vi "Full Force Test.vi"(8 "error in (no error)":errorcluster, 10 "Model in":refnum<class "Model.lvclass">, 11 "Test Actuator State in":refnum<class "Test Actuator State.lvclass">) -> (0 "error out":errorcluster, 2 "Model out":refnum<class "Model.lvclass">, 3 "Test Actuator State out":refnum<class "Test Actuator State.lvclass">)   [LabVIEW 2015, in "Test Actuator State.lvclass"]
uses:
  Test Actuator State.lvclass
  Model/Model/Model.lvclass
  Model/Model/Model.lvclass/Model.ctl
  Typedefs/ActuatorSetPoints.ctl
  Typedefs/FAMT Typedefs.lvlib
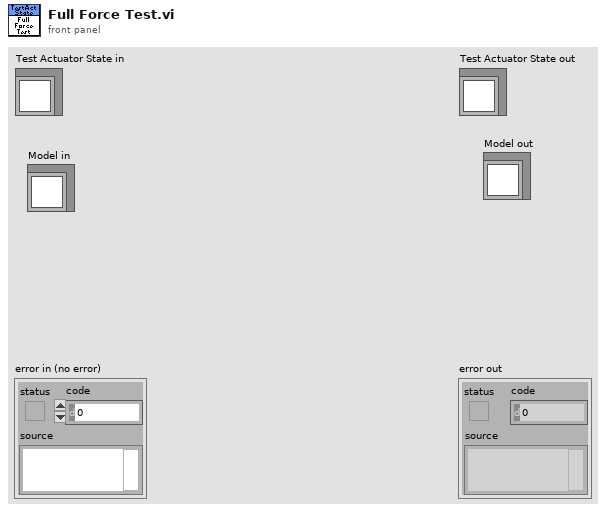
[diagram p1: front panel]
types:
  T1 = typedef "FAMT Typedefs.lvlib/FullForceScanSettings.ctl" = cluster{"Axial Force 1":dbl, "Lateral Force 1":dbl, "Axial Force 2":dbl, "Lateral Force 2":dbl, "Axial Force 3":dbl, "Lateral Force 3":dbl, "Axial Force 4":dbl, "Lateral Force 4":dbl, "Sample Time":dbl, "Process Time":dbl, "Tolerance %":dbl}
  T2 = cluster{"Axial Force 1":dbl, "Lateral Force 1":dbl}
  T3 = cluster{"Axial Force 2":dbl, "Lateral Force 2":dbl}
  T4 = cluster{"Axial Force 3":dbl, "Lateral Force 3":dbl}
  T5 = cluster{"Axial Force 4":dbl, "Lateral Force 4":dbl}
  T6 = cluster{"Axial Force 4":dbl, "Lateral Force 4":dbl}[]
  T7 = typedef "FAMT Typedefs.lvlib/ActuatorSetPoints.ctl" = cluster{"Axial Force":dbl, "Lateral Force":dbl, "FC1 Force":dbl, "FC2 Force":dbl}
  T8 = typedef "FAMT Typedefs.lvlib/ActuatorData.ctl" = cluster{"Timestamp":dbl, "Axial Force":dbl, "Lateral Force":dbl, "FC1 Force":dbl, "FC2 Force":dbl, "Lateral Push Pressure":dbl, "Lateral Pull Pressure":dbl, "Axial Push Pressure":dbl, "Axial Pull Pressure":dbl}
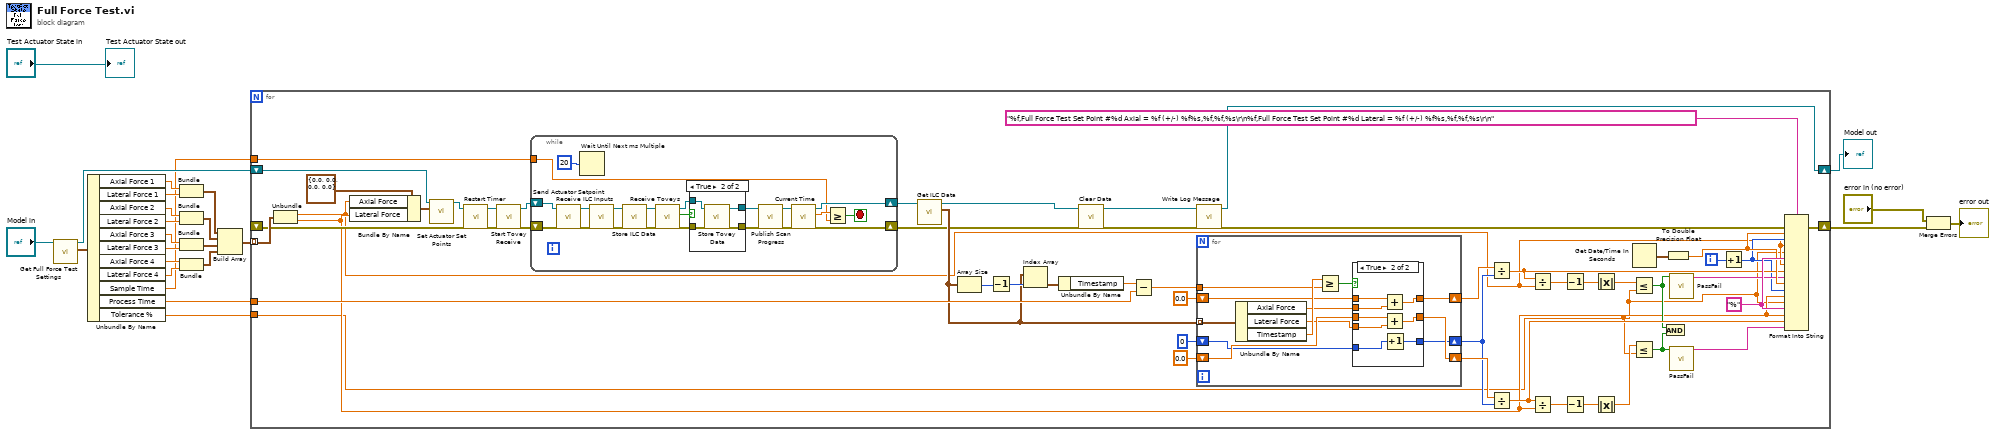
[diagram p0: block diagram]
diagram:
  n1 = call "Get Full Force Test Settings.vi"("Model in"="Model in") -> ("Full Force Test Settings"=w22:T1, "Model out"=w8:refnum<class "Model.lvclass">)  [unwired: 9 in]
  n2 = Unbundle By Name(w22) -> ("Axial Force 1"=w21:dbl, "Lateral Force 1"=w20:dbl, "Axial Force 2"=w18:dbl, "Lateral Force 2"=w17:dbl, "Axial Force 3"=w15:dbl, "Lateral Force 3"=w14:dbl, "Axial Force 4"=w12:dbl, "Lateral Force 4"=w11:dbl, "Sample Time"=w7:dbl, "Process Time"=w6:dbl, "Tolerance %"=w5:dbl)
  n3 = Bundle("Axial Force 1"=w21, "Lateral Force 1"=w20) -> (w19:T2)  [unwired: 1 in]
  n4 = Bundle("Axial Force 2"=w18, "Lateral Force 2"=w17) -> (w16:T3)  [unwired: 1 in]
  n5 = Bundle("Axial Force 3"=w15, "Lateral Force 3"=w14) -> (w13:T4)  [unwired: 1 in]
  n6 = Bundle("Axial Force 4"=w12, "Lateral Force 4"=w11) -> (w10:T5)  [unwired: 1 in]
  n7 = Build Array(w19, w16, w13, w10) -> (w9:T6)
  n8 = for {
    tunnel: w9 -> [w76] mode=indexing
    shift-right: [w49] -> w2
    shift-left: w8 -> [w75]
    tunnel: w7 -> [w74]
    tunnel: w6 -> [w68]
    tunnel: w5 -> [w31]
    shift-right: [w36] -> w1
    shift-left: _ -> [w51]
    i -> [w35]
    w45 = "%"
    n9 = Unbundle(w76) -> ("Axial Force 4"=w32:dbl, "Lateral Force 4"=w33:dbl)
    n10 = Bundle By Name(cluster=T7 {"Axial Force"=0.0, "Lateral Force"=0.0, "FC1 Force"=0.0, "FC2 Force"=0.0} ("Actuator Set Points"), "Axial Force"=w32, "Lateral Force"=w33) -> (w25:T7)
    n11 = call "Set Actuator Set Points.vi"("Actuator Set Points"=w25, "Model in"=w75) -> ("Model out"=w26:refnum<class "Model.lvclass">)  [unwired: 9 in]
    n12 = call "Restart Timer.vi"("error in (no error)"=w51, "Model in"=w26) -> ("error out"=w29:errorcluster, "Model out"=w30:refnum<class "Model.lvclass">)  [unwired: 8 in]
    n13 = call "Start Tovey Receive.vi"("error in (no error)"=w29, "Model in"=w30) -> ("error out"=w27:errorcluster, "Model out"=w28:refnum<class "Model.lvclass">)  [unwired: 8 in]
    n14 = while {
      shift-right: [w114] -> w73
      shift-left: w28 -> [w120]
      shift-right: [w113] -> w52
      shift-left: w27 -> [w117]
      tunnel: w74 -> [w111]
      stop <- w110 stop-if-true
      n15 = call "Send Actuator Setpoint.vi"("error in (no error)"=w117, "Model in"=w120) -> ("error out"=w116:errorcluster, "Model out"=w119:refnum<class "Model.lvclass">)  [unwired: 8 in]
      n16 = Wait Until Next ms Multiple(millisecond multiple=u32 20) -> ()  [unwired: 1 out]
      n17 = call "Receive ILC Inputs.vi"("error in (no error)"=w116, "Model in"=w119) -> ("error out"=w115:errorcluster, "Model out"=w118:refnum<class "Model.lvclass">)  [unwired: 8 in]
      n18 = call "Store ILC Data.vi"("error in (no error)"=w115, "Model in"=w118) -> ("error out"=w108:errorcluster, "Model out"=w109:refnum<class "Model.lvclass">)  [unwired: 8 in]
      n19 = call "Receive Toveys.vi"("error in (no error)"=w108, "Model in"=w109) -> ("error out"=w106:errorcluster, "Data Received"=w105:bool, "Model out"=w107:refnum<class "Model.lvclass">)  [unwired: 7 in]
      n20 = case shown="True" w105 {
        tunnel: w107 -> [w123 w127]
        tunnel: w106 -> [w122 w126]
        tunnel: [w122 w125] -> w101
        tunnel: [w123 w124] -> w104
        frame False {
        }
        frame True {
          n21 = call "Store Tovey Data.vi"("error in (no error)"=w126, "Model in"=w127) -> ("error out"=w125:errorcluster, "Model out"=w124:refnum<class "Model.lvclass">)  [unwired: 8 in]
        }
      }
      n22 = call "Publish Scan Progress.vi"("error in (no error)"=w101, "Model in"=w104) -> ("error out"=w102:errorcluster, "Model out"=w103:refnum<class "Model.lvclass">)  [unwired: 8 in]
      n23 = call "Current Time.vi"("error in (no error)"=w102, "Model in"=w103) -> ("error out"=w113:errorcluster, "Time"=w112:dbl, "Model out"=w114:refnum<class "Model.lvclass">)  [unwired: 7 in]
      n24 = Greater Or Equal?(x=w112, y=w111) -> (x >= y?=w110:bool)
    }
    n25 = call "Get ILC Data.vi"("Model in"=w73) -> ("ILCData"=w67:T8[], "Model out"=w53:refnum<class "Model.lvclass">)  [unwired: 9 in]
    n26 = Array Size(array=w67) -> (size(s)=w72:i32)
    n27 = Decrement(x=w72) -> (x-1=w71:i32)
    n28 = Index Array(array=w67, index=w71) -> (element=w70:T8)
    n29 = Unbundle By Name(w70) -> ("Timestamp"=w69:dbl)
    n30 = call "Clear Data.vi"("error in (no error)"=w52, "Model in"=w53) -> ("error out"=w48:errorcluster, "Model out"=w50:refnum<class "Model.lvclass">)  [unwired: 8 in]
    n31 = Subtract(x=w69, y=w68) -> (x-y=w66:dbl)
    n32 = call "Write Log Message.vi"("error in (no error)"=w48, "Model in"=w50) -> ("error out"=w37:errorcluster, "Model out"=w49:refnum<class "Model.lvclass">)  [unwired: 8 in]
    n33 = for {
      tunnel: w67 -> [w89] mode=indexing
      tunnel: w66 -> [w87]
      shift-right: [w84] -> w62
      shift-left: 0.0 -> [w86]
      shift-right: [w81] -> w61
      shift-left: 0.0 -> [w83]
      shift-right: [w78] -> w60
      shift-left: 0 -> [w79]
      n34 = Unbundle By Name(w89) -> ("Axial Force"=w85:dbl, "Lateral Force"=w82:dbl, "Timestamp"=w88:dbl)
      n35 = Greater Or Equal?(x=w88, y=w87) -> (x >= y?=w80:bool)
      n36 = case shown="True" w80 {
        tunnel: w86 -> [w91 w100]
        tunnel: w85 -> [_ w99]
        tunnel: [w91 w98] -> w84
        tunnel: w83 -> [w92 w97]
        tunnel: w82 -> [_ w96]
        tunnel: [w92 w95] -> w81
        tunnel: w79 -> [w90 w94]
        tunnel: [w90 w93] -> w78
        frame False {
        }
        frame True {
          n37 = Add(x=w100, y=w99) -> (x+y=w98:dbl)
          n38 = Add(x=w97, y=w96) -> (x+y=w95:dbl)
          n39 = Increment(x=w94) -> (x+1=w93:i32)
        }
      }
    }
    n40 = Divide(x=w62, y=w60) -> (x/y=w43:dbl)
    n41 = Divide(x=w61, y=w60) -> (x/y=w42:dbl)
    n42 = Divide(x=w43, y=w32) -> (x/y=w59:dbl)
    n43 = Divide(x=w42, y=w33) -> (x/y=w58:dbl)
    n44 = Decrement(x=w59) -> (x-1=w57:dbl)
    n45 = Decrement(x=w58) -> (x-1=w56:dbl)
    n46 = Absolute Value(x=w57) -> (abs(x)=w55:dbl)
    n47 = Absolute Value(x=w56) -> (abs(x)=w54:dbl)
    n48 = Less Or Equal?(x=w55, y=w31) -> (x <= y?=w41:bool)
    n49 = Less Or Equal?(x=w54, y=w31) -> (x <= y?=w39:bool)
    n50 = Get Date/Time In Seconds() -> (seconds since 1Jan1904=w46:timestamp)
    n51 = And(x=w41, y=w39) -> ()  [unwired: 1 out]
    n52 = To Double Precision Float(number=w46) -> (double precision float=w44:dbl)
    n53 = call "PassFail.vi"("Pass?"=w41) -> ("Result"=w40:string)  [unwired: 10 in]
    n54 = call "PassFail.vi"("Pass?"=w39) -> ("Result"=w38:string)  [unwired: 10 in]
    n55 = Increment(x=w35) -> (x+1=w34:i32)
    n56 = Format Into String(format string="%f,Full Force Test Set Point #%d Axial = %f (+/-) %f%s,%f,%f,%s\r\n%f,Full Force Test Set Point #%d Lateral = %f (+/-) %f%s,%f,%f,%s\r\n", error in=w37, w44, w34, w32, w31, w45, w32, w43, w40, w44, w34, w33, w31, w45, w33, w42, w38) -> (error out=w36:errorcluster)  [unwired: 1 in, 1 out]
  }
  "Model out" <- w2
  n57 = Merge Errors("error in (no error)", w1) -> (→"error out":errorcluster)
  "Test Actuator State out" <- "Test Actuator State in"
